vi "M1M3Support.vi"   [LabVIEW 2016]
uses:
  Common_FPGA_Timestamp/DataTypes/TimestampSettings.ctl
  Common_FPGA_HealthAndStatus/DataTypes/HealthAndStatusSettings.ctl
  Common_FPGA_HealthAndStatus/DataTypes/HealthAndStatusFIFOCopySettings.ctl
  Common_FPGA_Modbus/DataTypes/ModbusPortSettings.ctl
  Common_FPGA_T7Inclinometer/DataTypes/T7InclinometerSettings.ctl
  Common_FPGA_SerialASCII/DataTypes/SerialASCIISettings.ctl
  Common_FPGA_DIOSerial/DataTypes/DIOSerialPortSettings.ctl
  <vilib>/rvi/Emulation/niFpgaGetClockAttributes.vi
  <vilib>/rvi/Emulation/niFpgaSctlEmulationGetInTimedLoop.vi
  <vilib>/rvi/Emulation/niFpgaEmulationReportErrorSimple.vi
  <vilib>/rvi/eio/common/nirviEmuTemplateMethod_errors.vi
  <vilib>/rvi/Emulation/niFpgaCriticalErrorInLSC.vi
  <vilib>/rvi/Emulation/niFpgaEmulationIsFPGAContextNoSignature.vi
  <vilib>/rvi/DataTransferAndStorage/Container/Common/niFpgaContainerGetUniqueNameForEmu.vi
  <vilib>/rvi/Memory/Memory_Emulation/niFpgaMemoryEmulationCacheClearOnFirstRun.vi
  <vilib>/rvi/Memory/Memory_Emulation/nirvimemoryEmulationManagerCache_MakeExclusive.vi
  <vilib>/rvi/Memory/Memory_Emulation/niFpgaMemoryEmulationValidateCache.vi
  <vilib>/rvi/Memory/Memory_Emulation/nirvimemoryEmulationManagerCache_InsertValue.vi
  <vilib>/Utility/error.llb/Clear Errors.vi
  <vilib>/rvi/Memory/Memory_Emulation/nirvimemoryEmulationManagerCache_ReleaseExclusive.vi
  <vilib>/rvi/Memory/Memory_Emulation/nirvimemoryEmulationManagerCache_GetValue.vi
  <vilib>/rvi/Memory/Memory_Emulation/nirvimemoryEmulationManagerCache_SetValue.vi
  <vilib>/rvi/Emulation/niFpgaProcessEmulError.vi
  <vilib>/rvi/errors/niFpgaSetErrorForExecOnDevCompSimple.vi
  <vilib>/rvi/eio/common/nirviEmuReportErrorAndStop.vi
  <vilib>/rvi/FIFO/Fifo_Resource/nirvififoEmulationSetSize.vi
  <vilib>/rvi/FIFO/Fifo_Resource/nirviFifoEmulationQueueMgr.vi
  <instcachedir>/0/nirviFifoEmulationQueueMgr_E5CAEC123FF24DC58D834DCA3CDAA9B5.lvgen/nirviFifoEmulationQueueMgr_E5CAEC123FF24DC58D834DCA3CDAA9B5_007.vi
  <vilib>/rvi/FIFO/Fifo_Resource/nirvififoEmulationCreateLock.vi
  <vilib>/rvi/FIFO/Fifo_Resource/nirvififoEmulationObtainLock.vi
  <vilib>/rvi/FIFO/Fifo_Resource/nirvififoEmulationReleaseLock.vi
  <vilib>/rvi/occurrence/nirviWaitOnOccurrenceBase.vi
  <vilib>/rvi/errors/nirviReportUnexpectedCaseInternalError.vi
  <vilib>/rvi/errors/nirviReportUnexpectedCaseInternalError (U32).vi
  <vilib>/eio/EIOMethodNode/EIOMethodNode.xnode
  <vilib>/rvi/DataTransferAndStorage/Container/XNode/niFpgaContainer.xnode
  <vilib>/rvi/DataTransferAndStorage/Register/Emulation/niFpgaRegisterEmulation.vi
  <vilib>/eio/EIONode/EIONode.xnode
  <vilib>/rvi/FIFO/Fifo_Resource/nirvififoEmulationRead.vi
  Common_FPGA_Timestamp/FPGATimestamp.lvlib
  Common_FPGA_HealthAndStatus/FPGAHealthAndStatus.lvlib
  Common_FPGA_Modbus/FPGAModbus.lvlib
  Common_FPGA_T7Inclinometer/FPGAT7Inclinometer.lvlib
  Common_FPGA_SerialASCII/FPGASerialASCII.lvlib
  Common_FPGA_DIOSerial/FPGADIOSerial.lvlib
types:
  T1 = typedef "FPGADIOSerial.lvlib/DIOSerialPortSettings.ctl" = cluster{"TxPort":refnum<k21>, "TxDataFIFO":refnum<k21>, "TxInternalDataFIFO":refnum<k21>, "TxHealthAndStatusFIFO":refnum<k21>, "RxPort":refnum<k21>, "RxDataFIFO":refnum<k21>, "RxHealthAndStatusFIFO":refnum<k21>, "WaitForRxFrameRegister":refnum<k21>, "BaseHealthAndStatusAddress":u32, "IRQAddress":u8, "TriggerIRQRegister":refnum<k21>, "SoftwareControlledTrigger":refnum<k21>, "TimestampRegister":refnum<k21>, "TxTimestampFIFO":refnum<k21>}
  T2 = typedef "FPGAHealthAndStatus.lvlib/HealthAndStatusFIFOCopySettings.ctl" = cluster{"InternalHealthAndStatusFIFO":refnum<k21>, "SourceHealthAndStatusFIFO":refnum<k21>}
  T3 = typedef "FPGASerialASCII.lvlib/SerialASCIISettings.ctl" = cluster{"SerialPort":refnum<k21>, "TxFIFO":refnum<k21>, "RxFIFO":refnum<k21>, "TimestampRegister":refnum<k21>, "Terminator":u8, "ReadTimeoutMs":i16}
  T4 = typedef "FPGAT7Inclinometer.lvlib/T7InclinometerSettings.ctl" = cluster{"SerialPort":refnum<k21>, "TimestampRegister":refnum<k21>, "TxFIFO":refnum<k21>, "RxFIFO":refnum<k21>}
  T5 = typedef "FPGAModbus.lvlib/ModbusPortSettings.ctl" = cluster{"TxPort":refnum<k21>, "TxDataFIFO":refnum<k21>, "TxInternalDataFIFO":refnum<k21>, "TxHealthAndStatusFIFO":refnum<k21>, "RxPort":refnum<k21>, "RxDataFIFO":refnum<k21>, "RxHealthAndStatusFIFO":refnum<k21>, "WaitForRxFrameRegister":refnum<k21>, "BaseHealthAndStatusAddress":u32, "IRQAddress":u8, "TriggerIRQRegister":refnum<k21>, "SoftwareControlledTrigger":refnum<k21>, "TimestampRegister":refnum<k21>, "TxTimestampFIFO":refnum<k21>}
  T6 = typedef "FPGAHealthAndStatus.lvlib/HealthAndStatusSettings.ctl" = cluster{"InternalHealthAndStatusFIFO":refnum<k21>, "HealthAndStatusQueryFIFO":refnum<k21>, "HealthAndStatusResponseFIFO":refnum<k21>, "HealthAndStatusMemory":refnum<k21>, "MemorySize":i32}
  T7 = typedef "FPGATimestamp.lvlib/TimestampSettings.ctl" = cluster{"TimeSource":refnum<k21>, "TimeRegister":refnum<k21>, "IterationsPerMicrosecond":i16, "UpdateFIFO":refnum<k21>, "HealthAndStatusFIFO":refnum<k21>, "HealthAndStatusAddress":i16, "IterationsPerHealthAndStatusUpdate":i16}
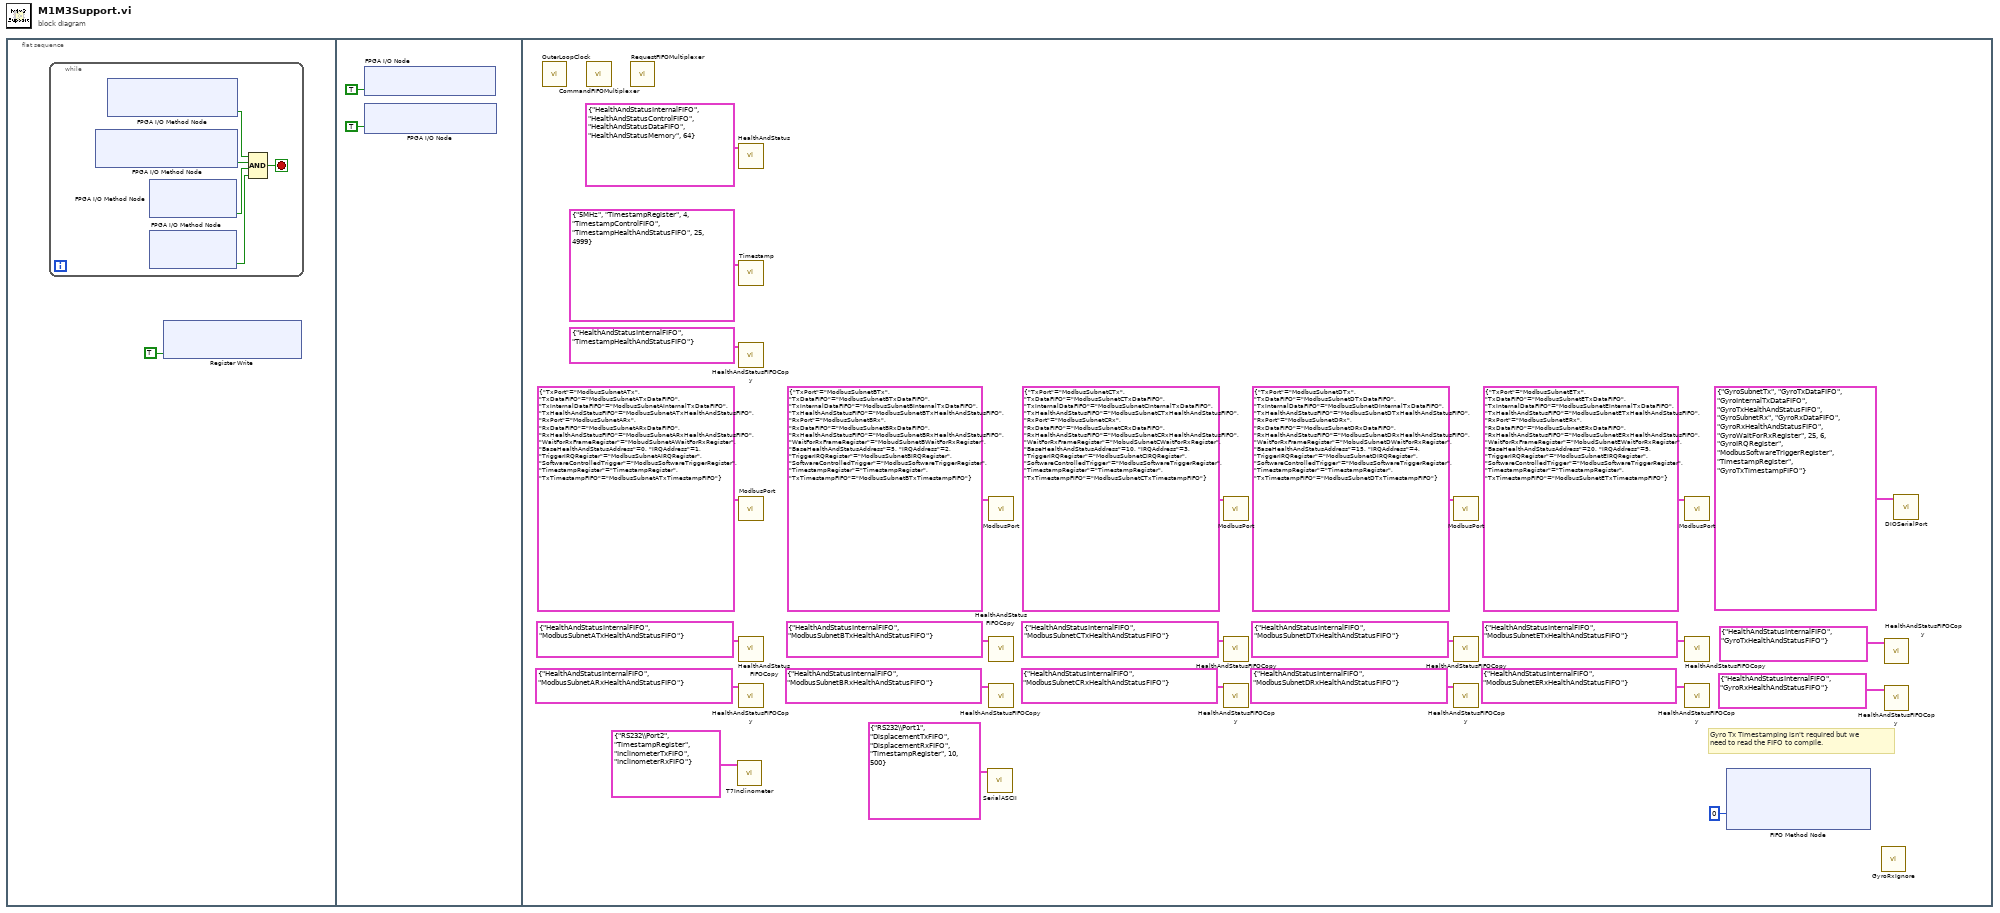
[diagram p0: block diagram]
diagram:
  n1 = flat-sequence {
    frame #0 {
      n2 = while {
        stop <- w2 stop-if-true
        n3 = xnode "FPGA I/O Method Node"() -> ("Ready"=w5:bool)  [unwired: 1 in, 1 out]
        n4 = xnode "FPGA I/O Method Node"() -> ("Ready"=w6:bool)  [unwired: 1 in, 1 out]
        n5 = xnode "FPGA I/O Method Node"() -> ("Ready"=w4:bool)  [unwired: 1 in, 1 out]
        n6 = xnode "FPGA I/O Method Node"() -> ("Ready"=w3:bool)  [unwired: 1 in, 1 out]
        n7 = Compound Arithmetic op=AND(w6, w5, w4, w3) -> (w2:bool)
      }
      n8 = xnode "Register Write"("Data"=TRUE) -> ()  [unwired: 1 in, 1 out]
    }
    frame #1 {
      n9 = xnode "FPGA I/O Node"("AccelerometerAB/Start"=TRUE) -> ()  [unwired: 1 in, 1 out]
      n10 = xnode "FPGA I/O Node"("AccelerometerCD/Start"=TRUE) -> ()  [unwired: 1 in, 1 out]
    }
    frame #2 {
      # "Gyro Tx Timestamping isn't required but we\nneed to read the FIFO to compile."
      n11 = call "OuterLoopClock.vi"() -> ()  [unwired: 12 in]
      n12 = call "CommandFIFOMultiplexer.vi"() -> ()  [unwired: 12 in]
      n13 = call "RequestFIFOMultiplexer.vi"() -> ()  [unwired: 12 in]
      n14 = call "T7Inclinometer.vi"("T7InclinometerSettings"=T4 {"SerialPort"="RS232\\Port2", "TimestampRegister"="TimestampRegister", "TxFIFO"="InclinometerTxFIFO", "RxFIFO"="InclinometerRxFIFO"}) -> ()  [unwired: 11 in]
      n15 = call "HealthAndStatus.vi"("HealthAndStatusSettings"=T6 {"InternalHealthAndStatusFIFO"="HealthAndStatusInternalFIFO", "HealthAndStatusQueryFIFO"="HealthAndStatusControlFIFO", "HealthAndStatusResponseFIFO"="HealthAndStatusDataFIFO", "HealthAndStatusMemory"="HealthAndStatusMemory", "MemorySize"=64}) -> ()  [unwired: 11 in]
      n16 = call "Timestamp.vi"("TimestampSettings"=T7 {"TimeSource"="5MHz", "TimeRegister"="TimestampRegister", "IterationsPerMicrosecond"=4, "UpdateFIFO"="TimestampControlFIFO", "HealthAndStatusFIFO"="TimestampHealthAndStatusFIFO", "HealthAndStatusAddress"=25, "IterationsPerHealthAndStatusUpdate"=4999}) -> ()  [unwired: 11 in]
      n17 = call "HealthAndStatusFIFOCopy.vi"("HealthAndStatusSettingsFIFOCopySettings"=T2 {"InternalHealthAndStatusFIFO"="HealthAndStatusInternalFIFO", "SourceHealthAndStatusFIFO"="TimestampHealthAndStatusFIFO"}) -> ()  [unwired: 11 in]
      n18 = call "ModbusPort.vi"("ModbusPortSettings"=T5 {"TxPort"="ModbusSubnetATx", "TxDataFIFO"="ModbusSubnetATxDataFIFO", "TxInternalDataFIFO"="ModbusSubnetAInternalTxDataFIFO", "TxHealthAndStatusFIFO"="ModbusSubnetATxHealthAndStatusFIFO", "RxPort"="ModbusSubnetARx", "RxDataFIFO"="ModbusSubnetARxDataFIFO", "RxHealthAndStatusFIFO"="ModbusSubnetARxHealthAndStatusFIFO", "WaitForRxFrameRegister"="MobudSubnetAWaitForRxRegister", "BaseHealthAndStatusAddress"=0, "IRQAddress"=1, "TriggerIRQRegister"="ModbusSubnetAIRQRegister", "SoftwareControlledTrigger"="ModbusSoftwareTriggerRegister", "TimestampRegister"="TimestampRegister", "TxTimestampFIFO"="ModbusSubnetATxTimestampFIFO"}) -> ()  [unwired: 10 in]
      n19 = call "HealthAndStatusFIFOCopy.vi"("HealthAndStatusSettingsFIFOCopySettings"=T2 {"InternalHealthAndStatusFIFO"="HealthAndStatusInternalFIFO", "SourceHealthAndStatusFIFO"="ModbusSubnetATxHealthAndStatusFIFO"}) -> ()  [unwired: 11 in]
      n20 = call "HealthAndStatusFIFOCopy.vi"("HealthAndStatusSettingsFIFOCopySettings"=T2 {"InternalHealthAndStatusFIFO"="HealthAndStatusInternalFIFO", "SourceHealthAndStatusFIFO"="ModbusSubnetARxHealthAndStatusFIFO"}) -> ()  [unwired: 11 in]
      n21 = call "SerialASCII.vi"("SerialASCIISettings"=T3 {"SerialPort"="RS232\\Port1", "TxFIFO"="DisplacementTxFIFO", "RxFIFO"="DisplacementRxFIFO", "TimestampRegister"="TimestampRegister", "Terminator"=10, "ReadTimeoutMs"=500}) -> ()  [unwired: 11 in]
      n22 = call "ModbusPort.vi"("ModbusPortSettings"=T5 {"TxPort"="ModbusSubnetBTx", "TxDataFIFO"="ModbusSubnetBTxDataFIFO", "TxInternalDataFIFO"="ModbusSubnetBInternalTxDataFIFO", "TxHealthAndStatusFIFO"="ModbusSubnetBTxHealthAndStatusFIFO", "RxPort"="ModbusSubnetBRx", "RxDataFIFO"="ModbusSubnetBRxDataFIFO", "RxHealthAndStatusFIFO"="ModbusSubnetBRxHealthAndStatusFIFO", "WaitForRxFrameRegister"="MobudSubnetBWaitForRxRegister", "BaseHealthAndStatusAddress"=5, "IRQAddress"=2, "TriggerIRQRegister"="ModbusSubnetBIRQRegister", "SoftwareControlledTrigger"="ModbusSoftwareTriggerRegister", "TimestampRegister"="TimestampRegister", "TxTimestampFIFO"="ModbusSubnetBTxTimestampFIFO"}) -> ()  [unwired: 10 in]
      n23 = call "HealthAndStatusFIFOCopy.vi"("HealthAndStatusSettingsFIFOCopySettings"=T2 {"InternalHealthAndStatusFIFO"="HealthAndStatusInternalFIFO", "SourceHealthAndStatusFIFO"="ModbusSubnetBTxHealthAndStatusFIFO"}) -> ()  [unwired: 11 in]
      n24 = call "HealthAndStatusFIFOCopy.vi"("HealthAndStatusSettingsFIFOCopySettings"=T2 {"InternalHealthAndStatusFIFO"="HealthAndStatusInternalFIFO", "SourceHealthAndStatusFIFO"="ModbusSubnetBRxHealthAndStatusFIFO"}) -> ()  [unwired: 11 in]
      n25 = call "ModbusPort.vi"("ModbusPortSettings"=T5 {"TxPort"="ModbusSubnetCTx", "TxDataFIFO"="ModbusSubnetCTxDataFIFO", "TxInternalDataFIFO"="ModbusSubnetCInternalTxDataFIFO", "TxHealthAndStatusFIFO"="ModbusSubnetCTxHealthAndStatusFIFO", "RxPort"="ModbusSubnetCRx", "RxDataFIFO"="ModbusSubnetCRxDataFIFO", "RxHealthAndStatusFIFO"="ModbusSubnetCRxHealthAndStatusFIFO", "WaitForRxFrameRegister"="MobudSubnetCWaitForRxRegister", "BaseHealthAndStatusAddress"=10, "IRQAddress"=3, "TriggerIRQRegister"="ModbusSubnetCIRQRegister", "SoftwareControlledTrigger"="ModbusSoftwareTriggerRegister", "TimestampRegister"="TimestampRegister", "TxTimestampFIFO"="ModbusSubnetCTxTimestampFIFO"}) -> ()  [unwired: 10 in]
      n26 = call "HealthAndStatusFIFOCopy.vi"("HealthAndStatusSettingsFIFOCopySettings"=T2 {"InternalHealthAndStatusFIFO"="HealthAndStatusInternalFIFO", "SourceHealthAndStatusFIFO"="ModbusSubnetCTxHealthAndStatusFIFO"}) -> ()  [unwired: 11 in]
      n27 = call "HealthAndStatusFIFOCopy.vi"("HealthAndStatusSettingsFIFOCopySettings"=T2 {"InternalHealthAndStatusFIFO"="HealthAndStatusInternalFIFO", "SourceHealthAndStatusFIFO"="ModbusSubnetCRxHealthAndStatusFIFO"}) -> ()  [unwired: 11 in]
      n28 = call "ModbusPort.vi"("ModbusPortSettings"=T5 {"TxPort"="ModbusSubnetDTx", "TxDataFIFO"="ModbusSubnetDTxDataFIFO", "TxInternalDataFIFO"="ModbusSubnetDInternalTxDataFIFO", "TxHealthAndStatusFIFO"="ModbusSubnetDTxHealthAndStatusFIFO", "RxPort"="ModbusSubnetDRx", "RxDataFIFO"="ModbusSubnetDRxDataFIFO", "RxHealthAndStatusFIFO"="ModbusSubnetDRxHealthAndStatusFIFO", "WaitForRxFrameRegister"="MobudSubnetDWaitForRxRegister", "BaseHealthAndStatusAddress"=15, "IRQAddress"=4, "TriggerIRQRegister"="ModbusSubnetDIRQRegister", "SoftwareControlledTrigger"="ModbusSoftwareTriggerRegister", "TimestampRegister"="TimestampRegister", "TxTimestampFIFO"="ModbusSubnetDTxTimestampFIFO"}) -> ()  [unwired: 10 in]
      n29 = call "HealthAndStatusFIFOCopy.vi"("HealthAndStatusSettingsFIFOCopySettings"=T2 {"InternalHealthAndStatusFIFO"="HealthAndStatusInternalFIFO", "SourceHealthAndStatusFIFO"="ModbusSubnetDTxHealthAndStatusFIFO"}) -> ()  [unwired: 11 in]
      n30 = call "HealthAndStatusFIFOCopy.vi"("HealthAndStatusSettingsFIFOCopySettings"=T2 {"InternalHealthAndStatusFIFO"="HealthAndStatusInternalFIFO", "SourceHealthAndStatusFIFO"="ModbusSubnetDRxHealthAndStatusFIFO"}) -> ()  [unwired: 11 in]
      n31 = call "ModbusPort.vi"("ModbusPortSettings"=T5 {"TxPort"="ModbusSubnetETx", "TxDataFIFO"="ModbusSubnetETxDataFIFO", "TxInternalDataFIFO"="ModbusSubnetEInternalTxDataFIFO", "TxHealthAndStatusFIFO"="ModbusSubnetETxHealthAndStatusFIFO", "RxPort"="ModbusSubnetERx", "RxDataFIFO"="ModbusSubnetERxDataFIFO", "RxHealthAndStatusFIFO"="ModbusSubnetERxHealthAndStatusFIFO", "WaitForRxFrameRegister"="MobudSubnetEWaitForRxRegister", "BaseHealthAndStatusAddress"=20, "IRQAddress"=5, "TriggerIRQRegister"="ModbusSubnetEIRQRegister", "SoftwareControlledTrigger"="ModbusSoftwareTriggerRegister", "TimestampRegister"="TimestampRegister", "TxTimestampFIFO"="ModbusSubnetETxTimestampFIFO"}) -> ()  [unwired: 10 in]
      n32 = call "HealthAndStatusFIFOCopy.vi"("HealthAndStatusSettingsFIFOCopySettings"=T2 {"InternalHealthAndStatusFIFO"="HealthAndStatusInternalFIFO", "SourceHealthAndStatusFIFO"="ModbusSubnetETxHealthAndStatusFIFO"}) -> ()  [unwired: 11 in]
      n33 = call "HealthAndStatusFIFOCopy.vi"("HealthAndStatusSettingsFIFOCopySettings"=T2 {"InternalHealthAndStatusFIFO"="HealthAndStatusInternalFIFO", "SourceHealthAndStatusFIFO"="ModbusSubnetERxHealthAndStatusFIFO"}) -> ()  [unwired: 11 in]
      n34 = xnode ("FIFO Method Node")("Timeout"=0) -> ()  [unwired: 1 in, 3 out]
      n35 = call "GyroRxIgnore.vi"() -> ()  [unwired: 12 in]
      n36 = call "HealthAndStatusFIFOCopy.vi"("HealthAndStatusSettingsFIFOCopySettings"=T2 {"InternalHealthAndStatusFIFO"="HealthAndStatusInternalFIFO", "SourceHealthAndStatusFIFO"="GyroTxHealthAndStatusFIFO"}) -> ()  [unwired: 11 in]
      n37 = call "HealthAndStatusFIFOCopy.vi"("HealthAndStatusSettingsFIFOCopySettings"=T2 {"InternalHealthAndStatusFIFO"="HealthAndStatusInternalFIFO", "SourceHealthAndStatusFIFO"="GyroRxHealthAndStatusFIFO"}) -> ()  [unwired: 11 in]
      n38 = call "DIOSerialPort.vi"("DIOSerialPortSettings"=T1 {"TxPort"="GyroSubnetTx", "TxDataFIFO"="GyroTxDataFIFO", "TxInternalDataFIFO"="GyroInternalTxDataFIFO", "TxHealthAndStatusFIFO"="GyroTxHealthAndStatusFIFO", "RxPort"="GyroSubnetRx", "RxDataFIFO"="GyroRxDataFIFO", "RxHealthAndStatusFIFO"="GyroRxHealthAndStatusFIFO", "WaitForRxFrameRegister"="GyroWaitForRxRegister", "BaseHealthAndStatusAddress"=25, "IRQAddress"=6, "TriggerIRQRegister"="GyroIRQRegister", "SoftwareControlledTrigger"="ModbusSoftwareTriggerRegister", "TimestampRegister"="TimestampRegister", "TxTimestampFIFO"="GyroTxTimestampFIFO"}) -> ()  [unwired: 10 in]
    }
  }
